vi "Configure Measure Layer Trigger Link.vi"(4 "Enable Output Trigger (F: Disable)":bool, 5 "Measure Semi-sync Trigger Line (1: Line1)":i32(ring)=1 items=["Line1"=1, "Line2"=2, "Line3"=3, "Line4"=4, "Line5"=5, "Line6"=6], 6 "Measure Output Trigger Line (1: Line1)":i32(ring)=1 items=["Line1"=1, "Line2"=2, "Line3"=3, "Line4"=4, "Line5"=5, "Line6"=6], 7 "Measure Input Trigger Line (2: Line2)":i32(ring)=2 items=["Line1"=1, "Line2"=2, "Line3"=3, "Line4"=4, "Line5"=5, "Line6"=6], 8 "error in (no error)":errorcluster, 9 "Measure Trigger Link Mode (0: Asynchronous)":i32(ring) items=["Asynchronous", "Synchronous"], 10 "Measure Source Bypass (1: Acceptor)":i32(ring)=1 items=["Source", "Acceptor"], 11 "VISA resource name":refnum<visa-resource-name>) -> (0 "error out":errorcluster, 3 "VISA resource name out":refnum<visa-resource-name>)   [LabVIEW 2019, in "Keithley 6517.lvlib"]
doc: "Sets bypass, protocol, input trigger line , output trigger line and semi-sync trigger line for the Measure Layer (Trigger) of the trigger model.\n\n<B>Note:</B>\n(1)<B>Models 6517A, 6517B:</B> The trigger model consists of 3 layers, the Arm Layer, the Scan Layer (Arm2), and the Measure Layer (Trigger).\n(2)<B>Model 6514:</B> The trigger model consists of 2 layers: Arm Layer & Measure Layer (Trigger).s"
uses:
  Keithley 6517.lvlib
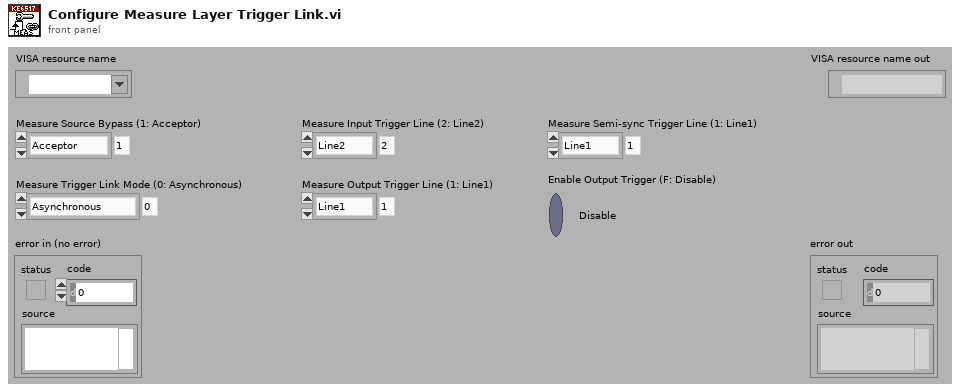
[diagram p1: front panel]
types:
  T1 = typedef "Keithley 6517.lvlib/Extended User Data.ctl" = cluster{"Instrument Model":i32}
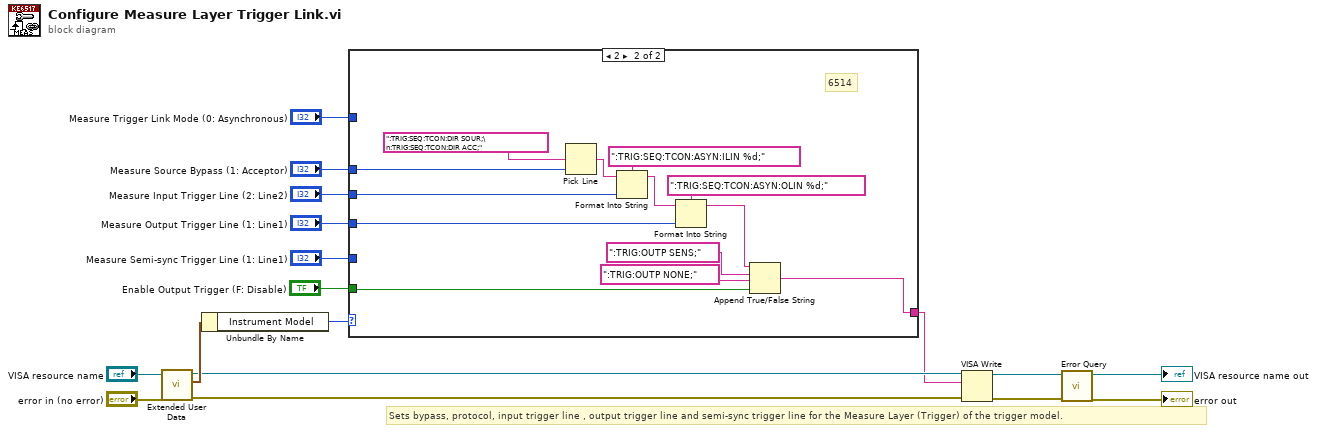
[diagram p0: block diagram]
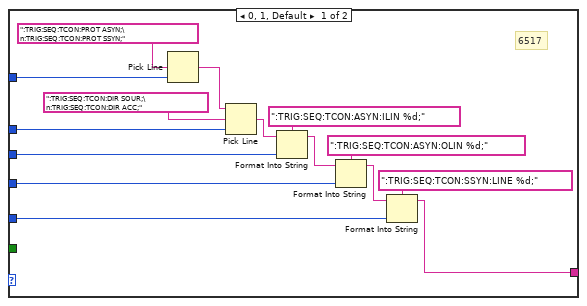
[diagram p2: hidden frame]
diagram:
  # "Sets bypass, protocol, input trigger line , output trigger line and semi-sync trigger line for the Measure Layer (Trigger) of the trigger model."
  n1 = call "Extended User Data.vi"("error in (no error)"="error in (no error)", "VISA resource name"="VISA resource name") -> ("error out"=w2:errorcluster, "User Data Out"=w5:T1, "VISA resource name out"=w3:refnum<visa-resource-name>)  [unwired: 7 in]
  n2 = Unbundle By Name(w5) -> ("Instrument Model"=w4:i32)
  n3 = case shown="2" w4 {
    tunnel: "Measure Input Trigger Line (2: Line2)" -> [w31 w44]
    tunnel: "Measure Output Trigger Line (1: Line1)" -> [w28 w41]
    tunnel: "Measure Semi-sync Trigger Line (1: Line1)" -> [w25 _]
    tunnel: "Measure Trigger Link Mode (0: Asynchronous)" -> [w24 _]
    tunnel: "Measure Source Bypass (1: Acceptor)" -> [w20 w39]
    tunnel: "Enable Output Trigger (F: Disable)" -> [_ w33]
    tunnel: [w18 w36] -> w1
    frame 0, 1, Default {
      # "6517"
      n4 = Pick Line(multi-line string=":TRIG:SEQ:TCON:PROT ASYN;\n:TRIG:SEQ:TCON:PROT SSYN;", line index=w24) -> (output string=w21:string)  [unwired: 1 in]
      n5 = Pick Line(string ("")=w21, multi-line string=":TRIG:SEQ:TCON:DIR SOUR;\n:TRIG:SEQ:TCON:DIR ACC;", line index=w20) -> (output string=w19:string)
      n6 = Format Into String(format string=":TRIG:SEQ:TCON:ASYN:ILIN %d;", initial string=w19, w31) -> (resulting string=w30:string)  [unwired: 1 in, 1 out]
      n7 = Format Into String(format string=":TRIG:SEQ:TCON:ASYN:OLIN %d;", initial string=w30, w28) -> (resulting string=w27:string)  [unwired: 1 in, 1 out]
      n8 = Format Into String(format string=":TRIG:SEQ:TCON:SSYN:LINE %d;", initial string=w27, w25) -> (resulting string=w18:string)  [unwired: 1 in, 1 out]
    }
    frame 2 {
      # "6514"
      n9 = Pick Line(multi-line string=":TRIG:SEQ:TCON:DIR SOUR;\n:TRIG:SEQ:TCON:DIR ACC;", line index=w39) -> (output string=w38:string)  [unwired: 1 in]
      n10 = Format Into String(format string=":TRIG:SEQ:TCON:ASYN:ILIN %d;", initial string=w38, w44) -> (resulting string=w43:string)  [unwired: 1 in, 1 out]
      n11 = Format Into String(format string=":TRIG:SEQ:TCON:ASYN:OLIN %d;", initial string=w43, w41) -> (resulting string=w37:string)  [unwired: 1 in, 1 out]
      n12 = Append True/False String(1:w33, 2:":TRIG:OUTP NONE;" ("true string"), 3:":TRIG:OUTP SENS;" ("true string"), 4:w37) -> (0:w36:string)
    }
  }
  n13 = VISA Write(VISA resource name=w3, write buffer=w1, error in (no error)=w2) -> (VISA resource name out=w14:refnum<visa-resource-name>, error out=w13:errorcluster)  [unwired: 1 out]
  n14 = call "Error Query.vi"("error in (no error)"=w13, "VISA resource name"=w14) -> ("error out"=→"error out":errorcluster, "VISA resource name out"=→"VISA resource name out":refnum<visa-resource-name>)  [unwired: 6 in, 2 out]
